vi "RFH-utility-average_common_format.vi"(10 "common array in":T1[](array[typedef])) -> (2 "Common Format":T1)   [LabVIEW 2020, in "RFH-Reflection_File_Handler.lvlib"]
uses:
  RFH-Reflection_File_Handler.lvlib
  RFH-common_data_format.ctl
panel:
  out "x = y?":bool
  out "Samples":i32
  out "Array 4":dbl[](array[numeric])
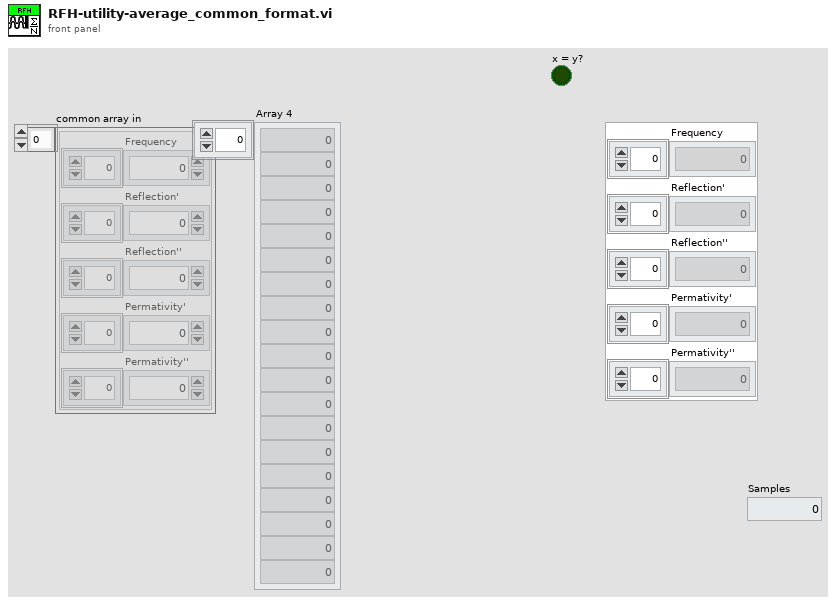
[diagram p1: front panel]
types:
  T1 = typedef "RFH-Reflection_File_Handler.lvlib/RFH-common_data_format.ctl" = cluster{"Frequency":dbl[], "Reflection'":dbl[], "Reflection''":dbl[], "Permativity'":dbl[], "Permativity''":dbl[]}
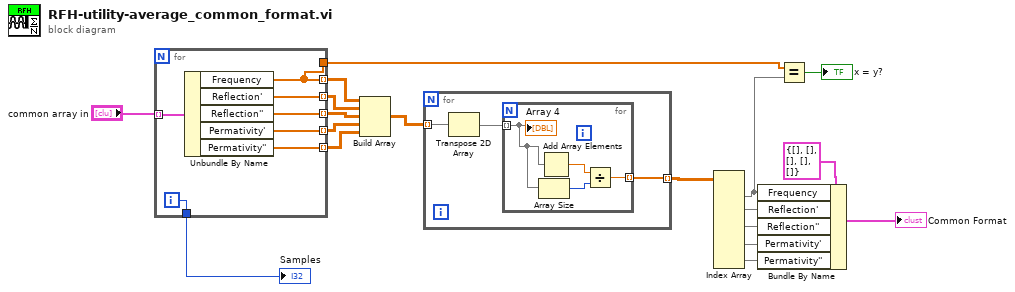
[diagram p0: block diagram]
diagram:
  n1 = for {
    tunnel: "common array in" -> [w25] mode=indexing
    tunnel: [w19] -> w18 mode=indexing
    tunnel: [w24] -> w17 mode=indexing
    tunnel: [w23] -> w16 mode=indexing
    tunnel: [w22] -> w15 mode=indexing
    tunnel: [w21] -> w14 mode=indexing
    tunnel: [w20] -> w12
    tunnel: [w19] -> w2
    i -> [w20]
    n2 = Unbundle By Name(w25) -> ("Frequency"=w19:dbl[], "Reflection'"=w24:dbl[], "Reflection''"=w23:dbl[], "Permativity'"=w22:dbl[], "Permativity''"=w21:dbl[])
  }
  "Samples" <- w12
  n3 = Build Array(w18, w17, w16, w15, w14) -> (w13:dbl[][][])
  n4 = for {
    tunnel: w13 -> [w28] mode=indexing
    tunnel: [w26] -> w10 mode=indexing
    n5 = Transpose 2D Array(2D array=w28) -> (transposed array=w27:dbl[][])
    n6 = for {
      tunnel: w27 -> [w30] mode=indexing
      tunnel: [w29] -> w26 mode=indexing
      n7 = Array Size(array=w30) -> (size(s)=w32:i32)
      n8 = Add Array Elements(numeric array=w30) -> (sum=w31:dbl)
      n9 = Divide(x=w31, y=w32) -> (x/y=w29:dbl)
      "Array 4" <- w30
    }
  }
  n10 = Index Array(array=w10) -> (element #1=w3:dbl[], element #2=w7:dbl[], element #3=w6:dbl[], element #4=w5:dbl[], element #5=w4:dbl[])  [unwired: 10 in]
  n11 = Bundle By Name(cluster=T1 {"Frequency"=[], "Reflection'"=[], "Reflection''"=[], "Permativity'"=[], "Permativity''"=[]} ("Common Format"), "Frequency"=w3, "Reflection'"=w7, "Reflection''"=w6, "Permativity'"=w5, "Permativity''"=w4) -> (→"Common Format":T1)
  n12 = Equal?(x=w2, y=w3) -> (x = y?=→"x = y?":bool)
